vi "encoders reading.vi"() -> ()   [LabVIEW 2015]
uses:
  <vilib>/myRIO/Common/Instrument Driver Framework/myRIO v1.0/Encoder/typedefs/Encoder Signal Mode.ctl
  <vilib>/myRIO/Instrument Drivers/Onboard IO/Encoder/typedefs/Encoder Reference.ctl
  <vilib>/myRIO/Common/Instrument Driver Framework/Utilities/typedefs/myRIO Generic Hardware Reference.ctl
  <vilib>/myRIO/Common/Instrument Driver Framework/Utilities/typedefs/Hardware Version Enum.ctl
  <vilib>/myRIO/Common/Instrument Driver Framework/Utilities/typedefs/myRIO v1.0 Reference.ctl
  <vilib>/myRIO/Common/Instrument Driver Framework/Utilities/typedefs/Generic FPGA Reference.ctl
  <vilib>/myRIO/Common/Instrument Driver Framework/myRIO v1.0/Encoder/typedefs/Encoder Channels Enum.ctl
  <vilib>/myRIO/Common/Instrument Driver Framework/myRIO v1.0/Encoder/typedefs/Encoder Configuration v1.0.ctl
  <vilib>/userdefined/High Color/nirio_resource_hc.ctl
  <vilib>/myRIO/Instrument Drivers/Onboard IO/DIO/typedefs/DIO Reference.ctl
  <vilib>/myRIO/Common/Instrument Driver Framework/myRIO v1.0/DIO/typedefs/DIO Channels List.ctl
  <vilib>/myRIO/Common/Instrument Driver Framework/myRIO v1.0/DIO/typedefs/DIO Channels Enum.ctl
  <vilib>/myRIO/Common/Instrument Driver Framework/Utilities/vis/Is FPGA Ref Available.vi
  <vilib>/myRIO/Common/Instrument Driver Framework/myRIO v1.0/Encoder/vis/myRIO v1.1 Open Encoder.vi
  <vilib>/myRIO/Instrument Drivers/Onboard IO/Encoder/vis/Read.vi
  <vilib>/myRIO/Common/Instrument Driver Framework/myRIO v1.0/DIO/vis/myRIO v1.1 Open DIO.vi
  <vilib>/myRIO/Instrument Drivers/Onboard IO/DIO/vis/Read.vi
  <vilib>/myRIO/Common/Instrument Driver Framework/Utilities/vis/Validate Channels.vi
  <vilib>/myRIO/Common/Instrument Driver Framework/myRIO v1.0/Encoder/vis/myRIO v1.0 Reserve Encoder.vi
  <vilib>/myRIO/Common/Instrument Driver Framework/myRIO v1.0/DIO/vis/myRIO v1.0 Reserve DIO.vi
  <vilib>/myRIO/Common/Instrument Driver Framework/myRIO v1.0/Encoder/vis/myRIO v1.0 Build MUX Configuration Encoder.vi
  <vilib>/myRIO/Common/Instrument Driver Framework/myRIO v1.0/Resource Manager/vis/myRIO v1.0 Reserve Channel List.vi
  <vilib>/myRIO/Common/Instrument Driver Framework/myRIO v1.0/DIO/vis/myRIO v1.0 Build MUX Configuration DIO.vi
  <vilib>/myRIO/Common/Instrument Driver Framework/myRIO v1.0/Resource Manager/vis/myRIO v1.0 Create Configuration List.vi
  <vilib>/myRIO/Common/Instrument Driver Framework/myRIO v1.0/Resource Manager/vis/myRIO v1.0 Reserve Channel.vi
  <vilib>/myRIO/Common/Instrument Driver Framework/myRIO v1.0/Resource Manager/vis/myRIO v1.0 Unreserve Channel.vi
  <vilib>/myRIO/Common/Instrument Driver Framework/myRIO v1.0/Resource Manager/vis/myRIO v1.0 Build Mutex Name.vi
  <vilib>/Utility/VariantDataType/GetNumericInfo.vi
  <vilib>/Utility/error.llb/Error Cluster From Error Code.vi
  <vilib>/myRIO/Common/Instrument Driver Framework/myRIO v1.0/myRIO v1.1 Open.vi
  <vilib>/myRIO/Common/Instrument Driver Framework/Utilities/vis/IO Manager.vi
  <vilib>/myRIO/Common/Instrument Driver Framework/Utilities/vis/Configuration Manager.vi
  <vilib>/myRIO/Common/Instrument Driver Framework/myRIO v1.0/Resource Manager/vis/myRIO v1.0 Configure IO.vi
  <vilib>/myRIO/Common/Instrument Driver Framework/myRIO v1.0/myRIO v1.0 Close.vi
  <vilib>/myRIO/Common/Instrument Driver Framework/myRIO v1.0/Encoder/vis/myRIO v1.0 Configure Encoder.vi
  <vilib>/myRIO/Common/Instrument Driver Framework/myRIO v1.0/Encoder/vis/myRIO v1.0 Read Encoder.vi
  <vilib>/myRIO/Common/Instrument Driver Framework/myRIO v1.0/DIO/vis/myRIO v1.0 Read DIO.vi
  <vilib>/myRIO/Express VI/Onboard IO/Encoder/Encoder Express VI.xnode
  <vilib>/myRIO/Instrument Drivers/Onboard IO/Encoder/vis/myRIO Encoder Open.xnode
  <vilib>/myRIO/Common/Instrument Driver Framework/myRIO v1.0/Encoder/typedefs/Encoder Count Direction Enum.ctl
  <vilib>/myRIO/Express VI/Onboard IO/DI/DI Express VI.xnode
  <vilib>/myRIO/Instrument Drivers/Onboard IO/DIO/vis/myRIO DIO Open.xnode
  <vilib>/myRIO/Instrument Drivers/Onboard IO/Encoder/Encoder.lvlib
  <vilib>/myRIO/Instrument Drivers/Onboard IO/DIO/DIO.lvlib
panel:
  in  "stop 3":bool
  out "Counter Value 4":i32
  out "Counter Direction 4":enum16{"Counting Up", "Counting Down"}(ring)
  out "Counter Value 3":i32
  out "Counter Direction 3":enum16{"Counting Up", "Counting Down"}(ring)
  in  "Motor Channel: (1 or 2)":u8=1
  in  "Stop (Brake or Coast)":string(combo)="Brake"
  in  "Select Channel":string(combo)="Motor 1"
  in  "Power (-100 to 100)\n0 = Stop/Brake\n-128 = Stop/Coast":i8(slide) scale=-100.0..100.0
  out "C/DIO7 (DIO7)":bool
  out "A/DIO4 (Pin 19)":bool
  out "A/DIO3 (Pin 17)":bool
  out "A/DIO2 (Pin 15)":bool
  out "A/DIO1 (Pin 13)":bool
  out "A/DIO0 (Pin 11)":bool
  in  "stop 2":bool
  out "Counter Direction 2":enum16{"Counting Up", "Counting Down"}(ring)
  out "Counter Value 2":i32
  in  "stop":bool
  out "Counter Direction":enum16{"Counting Up", "Counting Down"}(ring)
  out "Counter Value":i32
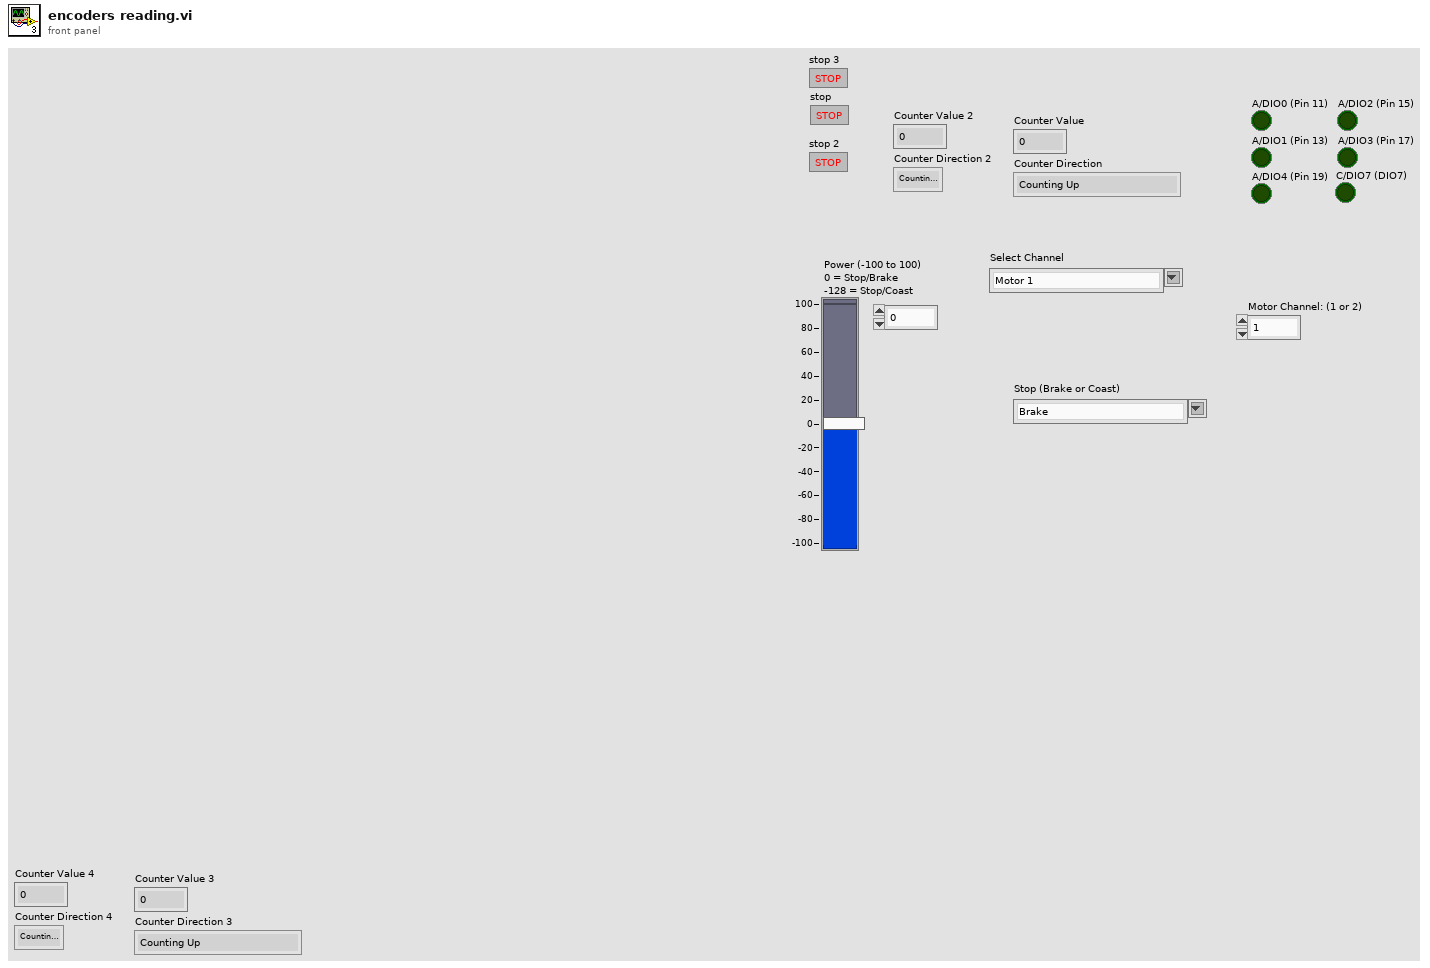
[diagram p1: front panel]
types:
  T1 = typedef "Encoder.lvlib/Encoder Reference.ctl" = cluster{"myRIO Reference":T2, "Encoder Channels Enum":T6}
  T2 = typedef "myRIO Generic Hardware Reference.ctl" = cluster{"myRIO Model":T3, "myRIO Hardware Reference":T4}
  T3 = typedef "Hardware Version Enum.ctl" = enum16{"Unknown", "myRIO-1900", "myRIO-1950", "roboRIO"}
  T4 = typedef "myRIO v1.0 Reference.ctl" = cluster{"Generic FPGA Reference":T5, "Allow multiple opens":bool}
  T5 = typedef "Generic FPGA Reference.ctl" = refnum<k20>
  T6 = typedef "Encoder Channels Enum.ctl" = enum16{"Not Connected", "C/ENC0", "C/ENC1", "A/ENC", "B/ENC", "DIO/ENC0", "DIO/ENC1", "DIO/ENC2", "DIO/ENC3", "DIO/ENC4"}
  T7 = typedef "Encoder Signal Mode.ctl" = enum16{"Quadrature phase signal", "Step and direction signal"}
  T8 = typedef "nirio_resource_hc.ctl" = tag
  T9 = typedef "Encoder Count Direction Enum.ctl" = enum16{"Counting Up", "Counting Down"}
  T10 = typedef "DIO.lvlib/DIO Reference.ctl" = cluster{"myRIO Reference":T2, "DIO Channels List":T11}
  T11 = typedef "DIO Channels List.ctl" = T12[]
  T12 = typedef "DIO Channels Enum.ctl" = enum16{"Not Connected", "C/DIO0", "C/DIO1", "C/DIO2", "C/DIO3", "C/DIO4", "C/DIO5", "C/DIO6", "C/DIO7", "A/DIO0", "A/DIO1", "A/DIO2", "A/DIO3", "A/DIO4", "A/DIO5", "A/DIO6", "A/DIO7", "A/DIO8", "A/DIO9", "A/DIO10", "A/DIO11", "A/DIO12", "A/DIO13", "A/DIO14", "A/DIO15", "B/DIO0", "B/DIO1", "B/DIO2", "B/DIO3", "B/DIO4", "B/DIO5", "B/DIO6", "B/DIO7", "B/DIO8", "B/DIO9", "B/DIO10", "B/DIO11", "B/DIO12", "B/DIO13", "B/DIO14", "B/DIO15", "LED0", "LED1", "LED2", "LED3", "Button0", "DIO/DIO0", "DIO/DIO1", "DIO/DIO2", "DIO/DIO3", "DIO/DIO4", "DIO/DIO5", "DIO/DIO6", "DIO/DIO7", "DIO/DIO8", "DIO/DIO9", "SPI/CS0", "SPI/CS1", "SPI/CS2", "SPI/CS3", "LED RADIO (Green)", "LED RADIO (Red)", "LED COMM (Green)", "LED COMM (Red)", "LED MODE (Green)", "LED MODE (Red)"}
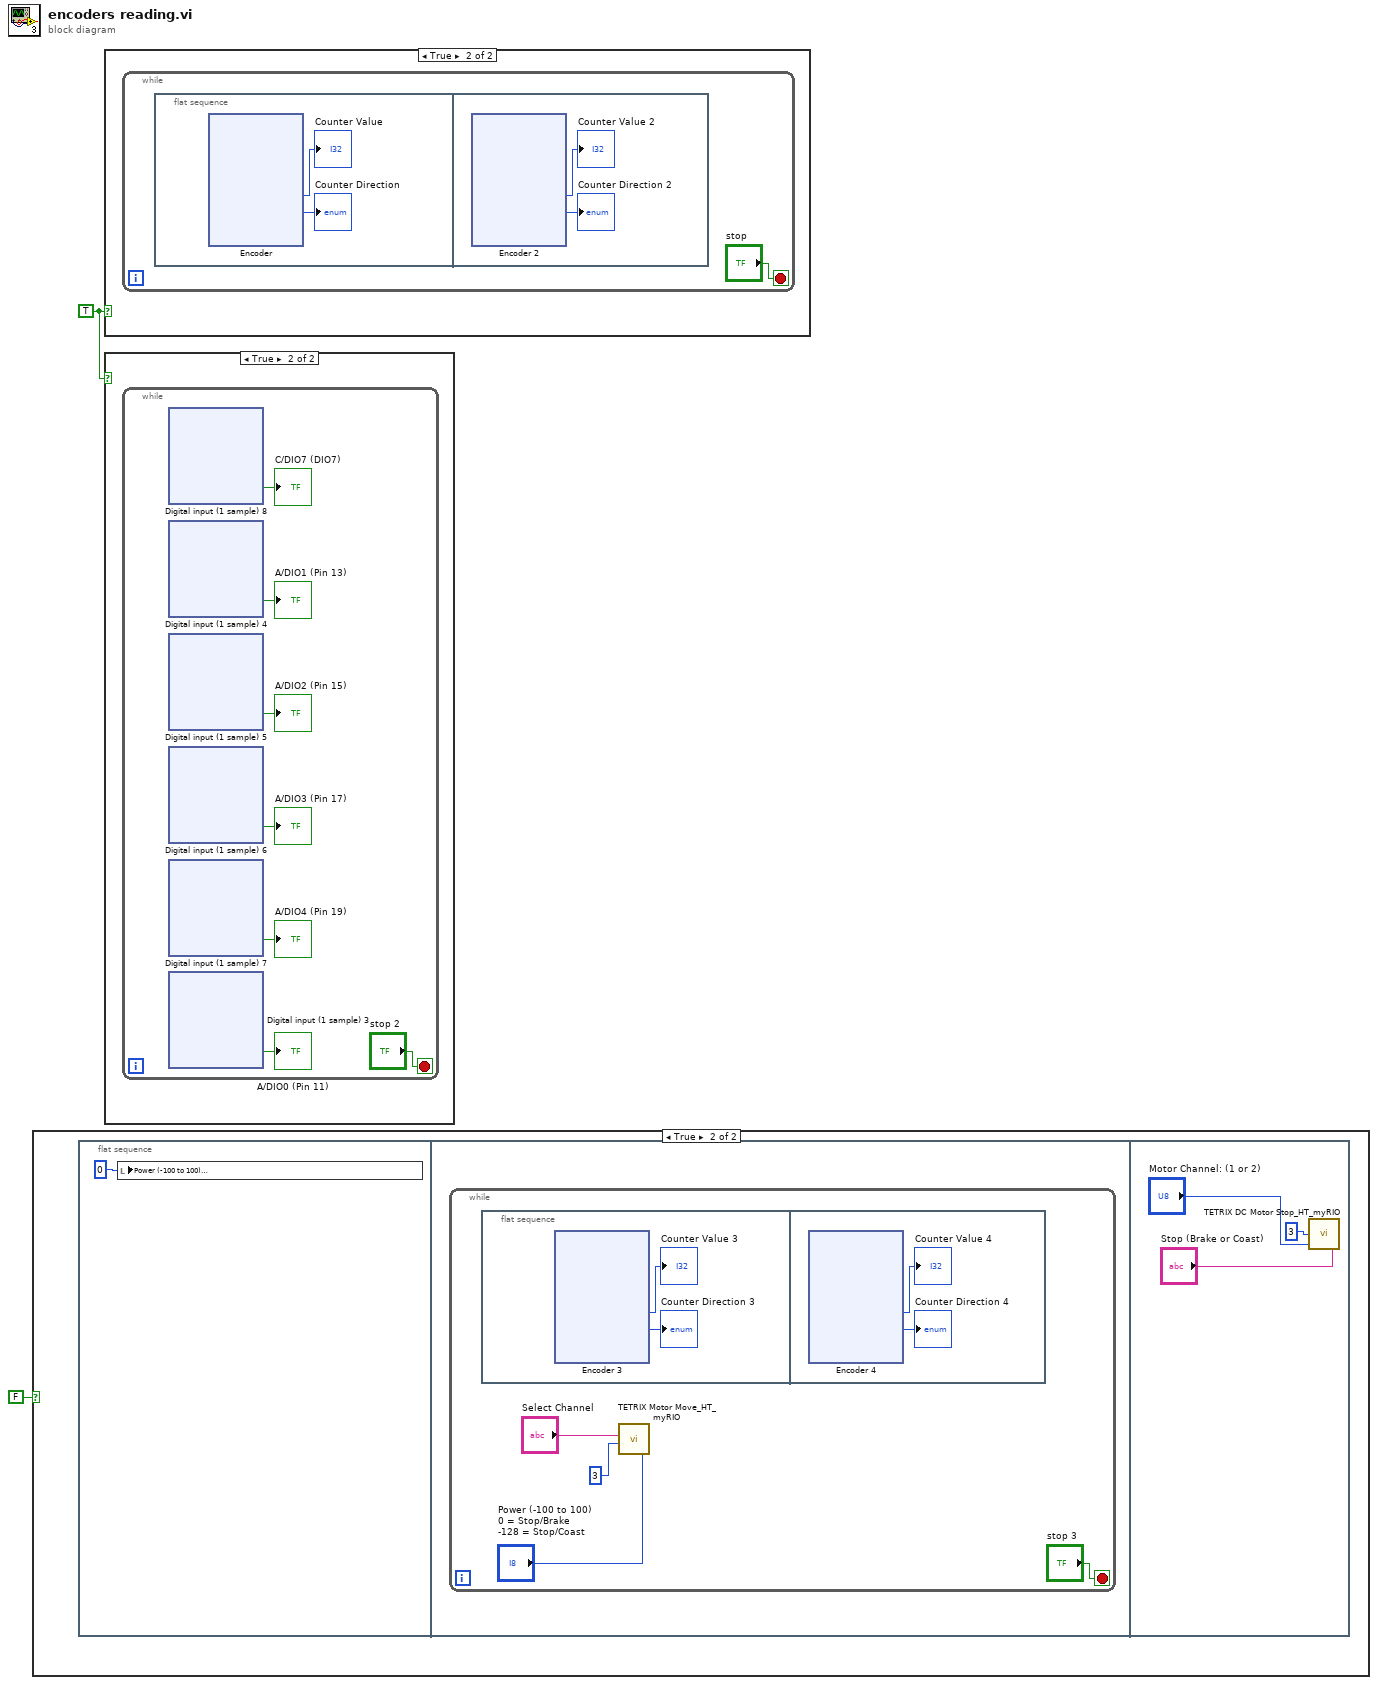
[diagram p0: block diagram]
diagram:
  w2 = TRUE
  n1 = case shown="True" FALSE {
    frame False {
    }
    frame True {
      n2 = flat-sequence {
        frame #0 {
          n3 = local write "Power (-100 to 100)\n0 = Stop/Brake\n-128 = Stop/Coast"(i8 0 ("Power (-100 to 100)\n0 = Stop/Brake\n-128 = Stop/Coast")) -> ()
        }
        frame #1 {
          n4 = while {
            stop <- "stop 3" stop-if-true
            n5 = flat-sequence {
              frame #0 {
                n6 = xnode "Encoder 3"() -> ("Counter Value"=→"Counter Value 3":i32, "Counter Direction"=→"Counter Direction 3":enum16{"Counting Up", "Counting Down"})  [unwired: 2 in, 2 out]
              }
              frame #1 {
                n7 = xnode "Encoder 4"() -> ("Counter Value"=→"Counter Value 4":i32, "Counter Direction"=→"Counter Direction 4":T9)  [unwired: 2 in, 2 out]
              }
            }
            n8 = call <vilib>:"TETRIX Motor Move_HT_myRIO.vi"("Power (-100 to 100)\n0 = Stop/Brake\n-128 = Stop/Coast"="Power (-100 to 100)\n0 = Stop/Brake\n-128 = Stop/Coast", "Controller Daisy Chain Position: 1 - 4"=u8 3, "Select Channel"="Select Channel") -> ()  [unwired: 4 in, 1 out]
          }
        }
        frame #2 {
          n9 = call <vilib>:"TETRIX DC Motor Stop_HT_myRIO.vi"("Stop (Brake or Coast)"="Stop (Brake or Coast)", "Motor Channel: (1 or 2)"="Motor Channel: (1 or 2)", "Controller Daisy Chain Position: 1 - 4"=u8 3) -> ()  [unwired: 1 in, 1 out]
        }
      }
    }
  }
  n10 = case shown="True" w2 {
    frame False {
    }
    frame True {
      n11 = while {
        stop <- "stop" stop-if-true
        n12 = flat-sequence {
          frame #0 {
            n13 = xnode "Encoder"() -> ("Counter Value"=→"Counter Value":i32, "Counter Direction"=→"Counter Direction":enum16{"Counting Up", "Counting Down"})  [unwired: 2 in, 2 out]
          }
          frame #1 {
            n14 = xnode "Encoder 2"() -> ("Counter Value"=→"Counter Value 2":i32, "Counter Direction"=→"Counter Direction 2":T9)  [unwired: 2 in, 2 out]
          }
        }
      }
    }
  }
  n15 = case shown="True" w2 {
    frame False {
    }
    frame True {
      n16 = while {
        stop <- "stop 2" stop-if-true
        n17 = xnode "Digital input (1 sample) 8"() -> ("C/DIO7 (DIO7)"=→"C/DIO7 (DIO7)":bool)  [unwired: 1 in, 1 out]
        n18 = xnode "Digital input (1 sample) 4"() -> ("A/DIO1 (Pin 13)"=→"A/DIO1 (Pin 13)":bool)  [unwired: 1 in, 1 out]
        n19 = xnode "Digital input (1 sample) 5"() -> ("A/DIO2 (Pin 15)"=→"A/DIO2 (Pin 15)":bool)  [unwired: 1 in, 1 out]
        n20 = xnode "Digital input (1 sample) 6"() -> ("A/DIO3 (Pin 17)"=→"A/DIO3 (Pin 17)":bool)  [unwired: 1 in, 1 out]
        n21 = xnode "Digital input (1 sample) 7"() -> ("A/DIO4 (Pin 19)"=→"A/DIO4 (Pin 19)":bool)  [unwired: 1 in, 1 out]
        n22 = xnode "Digital input (1 sample) 3"() -> ("A/DIO0 (Pin 11)"=→"A/DIO0 (Pin 11)":bool)  [unwired: 1 in, 1 out]
      }
    }
  }
